vi "Script Msg VI.vi"(6 "Name":string, 8 "error in":errorcluster, 9 "Ref.Msg VI":refnum<vi>, 10 "Conpane Map":T1(c390)) -> (0 "error out":errorcluster)   [LabVIEW 2021, in "_Msg Rescript.lvlib" / "_Msg Rescript.lvclass"]
uses:
  _Msg Rescript.lvclass
  <vilib>/Utility/traverseref.llb/TRef TravTarget.ctl
  _Msg Rescript.lvclass/_Msg Rescript.ctl
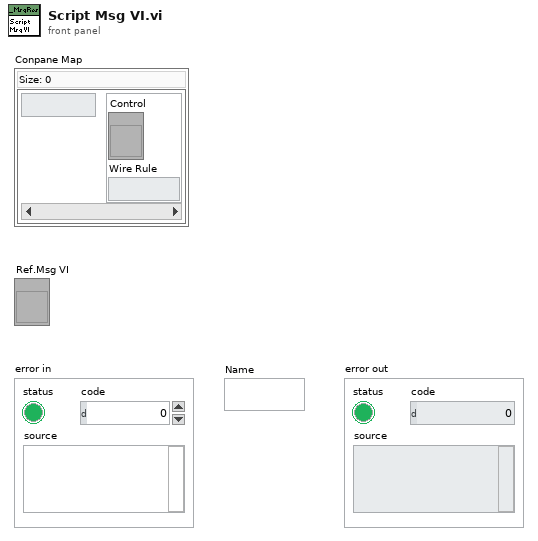
[diagram p1: front panel]
types:
  T1 = map{i32, cluster{"Control":refnum<vi>, "Wire Rule":enum16{"Invalid Wire Rule", "Required", "Recommended", "Optional", "Dynamic Dispatch"}}}
  T2 = typedef "TRef TravTarget.ctl" = enum16{"FP", "BD", "Other"}
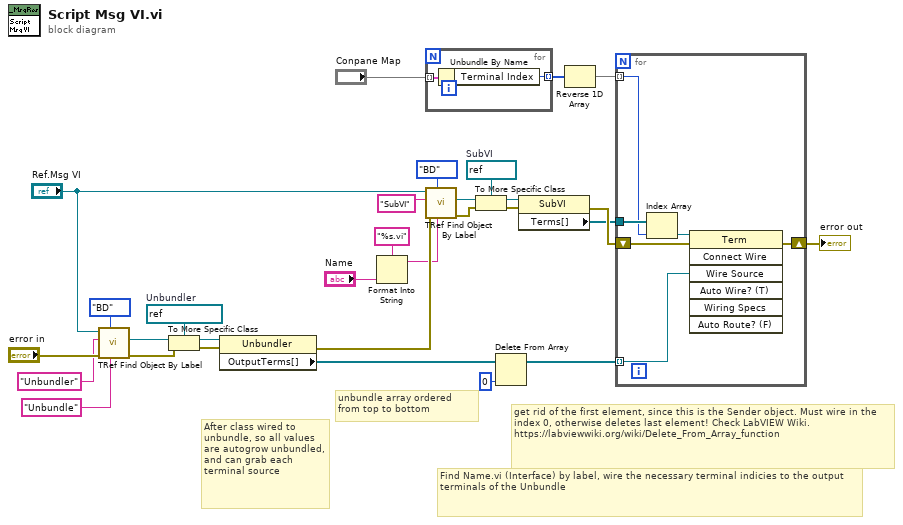
[diagram p0: block diagram]
diagram:
  w12 = refnum<vi> refnum  # Unbundler
  w29 = refnum<vi> refnum  # SubVI
  # "unbundle array ordered from top to bottom"
  # "get rid of the first element, since this is the Sender object. Must wire in the index 0, otherwise deletes last element! Check LabVIEW Wiki.\nhttps://labviewwiki.org/wiki/Delete_From_Array_function"
  # "After class wired to unbundle, so all values are autogrow unbundled, and can grab each terminal source"
  # "Find Name.vi (Interface) by label, wire the necessary terminal indicies to the output terminals of the Unbundle"
  n1 = call <vilib>:"TRef Find Object By Label.vi"("Label"="Unbundle", "Traverse Target"=TRef_TravTarget."BD", "error in (no error)"="error in", "Class Name"="Unbundler", "VI Ref"="Ref.Msg VI") -> ("error out"=w13:errorcluster, "Found Obj Ref"=w11:refnum<vi>)  [unwired: 3 in, 2 out]
  n2 = To More Specific Class(target class=w12, reference=w11, error in=w13) -> (specific class reference=w8:refnum<vi>, error out=w4:errorcluster)
  n3 = property class="Unbundler"(reference=w8, error in=w4) -> (error out=w19:errorcluster, "OutputTerms[]"=w3:refnum<vi>[])  [unwired: 1 out]
  n4 = Format Into String(format string="%s.vi", "Name") -> (resulting string=w14:string)  [unwired: 2 in, 1 out]
  n5 = for {
    tunnel: "Conpane Map" -> [w32] mode=indexing
    tunnel: [w31] -> w24 mode=indexing
    n6 = Unbundle By Name(w32) -> ("Terminal Index"=w31:i32)
  }
  n7 = call <vilib>:"TRef Find Object By Label.vi"("Label"=w14, "Traverse Target"=TRef_TravTarget."BD", "error in (no error)"=w19, "Class Name"="SubVI", "VI Ref"="Ref.Msg VI") -> ("error out"=w28:errorcluster, "Found Obj Ref"=w18:refnum<vi>)  [unwired: 3 in, 2 out]
  n8 = To More Specific Class(target class=w29, reference=w18, error in=w28) -> (specific class reference=w26:refnum<vi>, error out=w25:errorcluster)
  n9 = Delete From Array(array=w3, index=0) -> (array with subset deleted=w2:refnum<vi>[])  [unwired: 1 in, 1 out]
  n10 = property class="SubVI"(reference=w26, error in=w25) -> (error out=w23:errorcluster, "Terms[]"=w22:refnum<vi>[])  [unwired: 1 out]
  n11 = Reverse 1D Array(array=w24) -> (reversed array=w20:i32[])
  n12 = for {
    tunnel: w22 -> [w38]
    tunnel: w20 -> [w37] mode=indexing
    shift-right: [w34] -> w15
    shift-left: w23 -> [w35]
    tunnel: w2 -> [w33] mode=indexing
    n13 = Index Array(array=w38, index=w37) -> (element=w36:refnum<vi>)
    n14 = invoke class="Term" method="Connect Wire"(reference=w36, error in=w35, "Wire Source"=w33) -> (error out=w34:errorcluster)  [unwired: 4 in, 6 out]
  }
  "error out" <- w15
